vi "FTP File Control.vi"(7 "Comm":enum16{"Get", "Put"}(ring), 8 "에러 입력":errorcluster caption="에러 입력(에러 없음)", 9 "원격경로":string, 10 "로컬경로":path, 11 "TCP 네트워크 연결 입력":T2) -> (0 "에러 출력":errorcluster, 1 "파일존재?":bool, 2 "로컬경로 out":path, 3 "TCP 네트워크 연결 출력":T2, 5 "출력 클러스터":T1)   [LabVIEW 2020]
uses:
  <vilib>/FTP/ftp0.llb/FTP Session.ctl
  <vilib>/security/Message Digest/API/Instances/File/SHA-256 File Checksum.vi
  <vilib>/FTP/NI_FTP.lvlib
  <vilib>/security/Message Digest/API/NI_Message Digest API.lvlib
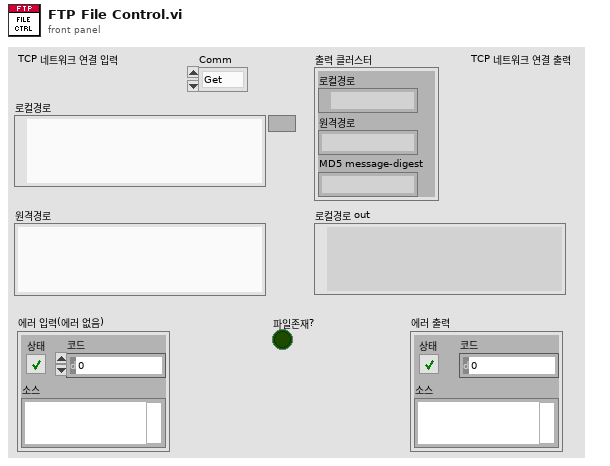
[diagram p1: front panel]
types:
  T1 = cluster{"로컬경로":path, "원격경로":string, "MD5 message-digest":string}
  T2 = typedef "NI_FTP.lvlib/FTP Session.ctl" = refnum<k5>
  T3 = cluster{"로컬경로":path, "원격경로":string, "digest":string}
  T4 = cluster{"원격경로":string, "로컬경로":path, "모두 대체? (거짓)":bool, string}
  T5 = cluster{"원격경로":string, "로컬경로":path, "모두 대체? (거짓)":bool, string}[]
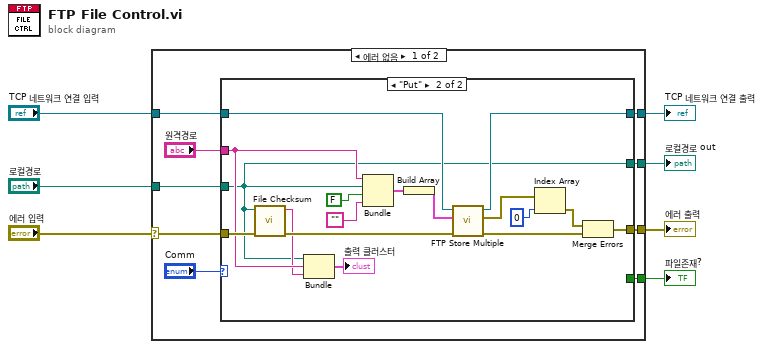
[diagram p0: block diagram]
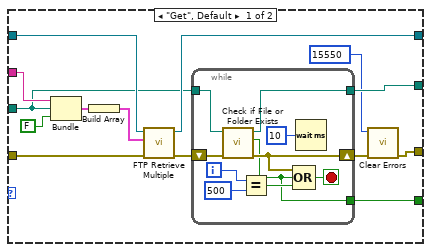
[diagram p2: hidden frame]
diagram:
  n1 = case shown="에러 없음" "에러 입력" {
    selector: "에러 입력" -> [w13 w60]
    tunnel: [w16 w59] -> w7
    tunnel: "TCP 네트워크 연결 입력" -> [w15 w59]
    tunnel: [w14 w60] -> w5
    tunnel: "로컬경로" -> [w11 w58]
    tunnel: [w9 w58] -> w2
    tunnel: [w8 _] -> w1
    frame No Error {
      n2 = case shown="\"Put\"" "Comm" {
        tunnel: [w23 w56] -> w16
        tunnel: w15 -> [w25 w55]
        tunnel: [w18 w47] -> w14
        tunnel: w13 -> [w27 w46]
        tunnel: "원격경로" -> [w26 w44]
        tunnel: w11 -> [w22 w41]
        tunnel: [w21 w41] -> w9
        tunnel: [w20 _] -> w8
        frame "Get", Default {
          n3 = Bundle("원격경로"=w26, "로컬경로"=w22, FALSE) -> (w30:cluster{"원격경로":string, "로컬경로":path, bool})  [unwired: 1 out]
          n4 = Build Array(w30) -> (w29:cluster{"원격경로":string, "로컬경로":path, bool}[])
          n5 = call <vilib>:"FTP Retrieve Multiple.vi"("error in (no error)"=w27, "file specifications"=w29, "ftp session"=w25) -> ("error out"=w24:errorcluster, "ftp session out"=w23:T2)  [unwired: 2 in, 5 out]
          n6 = while {
            shift-right: [w32] -> w19
            shift-left: w24 -> [w40]
            tunnel: w22 -> [w39]
            tunnel: [w34] -> w21
            tunnel: [w31] -> w20
            i -> [w37]
            stop <- w33 stop-if-true
            n7 = call <vilib>:"Check if File or Folder Exists.vi"("error in (no error)"=w40, "path"=w39) -> ("error out"=w32:errorcluster, "file or folder exists?"=w31:bool, "dup path"=w34:path)  [unwired: 7 in]
            n8 = Equal?(x=w37, y=500) -> (x = y?=w38:bool)
            n9 = Compound Arithmetic op=OR(w32, w31, w38) -> (w33:bool)
            n10 = Wait (ms)(milliseconds to wait=u32 10 ("대기 시간(ms)")) -> ()  [unwired: 1 out]
          }
          n11 = call <vilib>:"Clear Errors.vi"("error in (no error)"=w19, "specific error code to clear (0: all)"=15550) -> ("error out"=w18:errorcluster)  [unwired: 4 in, 1 out]
        }
        frame "Put" {
          n12 = call-poly <vilib>:"File Checksum.vi"("error in"=w46, "path"=w41) -> ("error out"=w45:errorcluster, "digest"=w43:string)  [unwired: 8 in]
          n13 = Bundle("로컬경로"=w41, "원격경로"=w44, "digest"=w43) -> (→"출력 클러스터":T3)  [unwired: 1 in]
          n14 = Bundle("원격경로"=w44, "로컬경로"=w41, "모두 대체? (거짓)"=FALSE, "") -> (w53:T4)  [unwired: 1 out]
          n15 = Build Array(w53) -> (w57:T5)
          n16 = call <vilib>:"FTP Store Multiple.vi"("error in (no error)"=w45, "file specifications"=w57, "ftp session"=w55) -> ("error out"=w48:errorcluster, "file errors"=w51:errorcluster[], "ftp session out"=w56:T2)  [unwired: 6 in]
          n17 = Index Array(array=w51, index=0 ("인덱스")) -> (element=w49:errorcluster)
          n18 = Merge Errors(w49, w48) -> (w47:errorcluster)
        }
      }
    }
    frame Error {
    }
  }
  "TCP 네트워크 연결 출력" <- w7
  "에러 출력" <- w5
  "파일존재?" <- w1
  "로컬경로 out" <- w2
